vi "Teleop.vi"(10 "Match Info":T1={"Autonomous Elapsed Seconds"=0.0, "TeleOp Elapsed Seconds"=0.0, "Disabled Elapsed Seconds"=0.0, "Visited Autonomous"=FALSE, "Visited TeleOp"=FALSE, "Visited Disabled"=FALSE, "Autonomous Settings"={"Autonomous Style"=enum."Independent", "VI Refnum"=refnum}}, 11 "Call Context":T2) -> ()   [LabVIEW 2012]
doc: "This VI is called for each TeleOp packet received from the DS where the robot is not disabled. It is often used to read from the joysticks and update I/O or to update setpoints for timed control loops. It should complete and return within 20 milliseconds or it may miss DS packets."
uses:
  <vilib>/Rock Robotics/WPI/DriverStation/WPI_DriverStationDerivedRobotMode.ctl
  <vilib>/Rock Robotics/WPI/DriverStation/WPI_DriverStationMatch Info.ctl
  BotStatus.vi
  Robot Global Data.vi
  <vilib>/Rock Robotics/WPI/Joystick/WPI_JoystickGetSetRefNum.vi
  <vilib>/Rock Robotics/WPI/RobotDrive/WPI_RobotDriveGetSetRefNum.vi
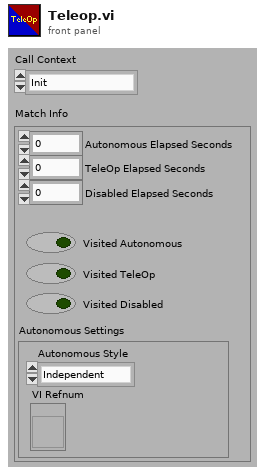
[diagram p1: front panel]
types:
  T1 = typedef "WPI_DriverStationMatch Info.ctl" = cluster{"Autonomous Elapsed Seconds":dbl, "TeleOp Elapsed Seconds":dbl, "Disabled Elapsed Seconds":dbl, "Visited Autonomous":bool, "Visited TeleOp":bool, "Visited Disabled":bool, "Autonomous Settings":cluster{"Autonomous Style":enum16{"Iterative", "Independent"}, "VI Refnum":refnum<vi>}}
  T2 = typedef "WPI_DriverStationDerivedRobotMode.ctl" = enum16{"Init", "Execute", "Stop"}
  T3 = typedef "WPI_JoystickDevRef.ctl" = cluster{"Device":T4}
  T4 = typedef "WPI_JoystickDeviceEnum.ctl" = enum16{"USB 1", "USB 2", "USB 3", "USB 4", "Kinect 1", "Kinect 2"}
  T5 = cluster{"Middle":bool, "InFlipper":bool, "Bottom":bool, "FlipperDown":bool, "Frizbee Counter":dbl}
  T6 = typedef "WPI_RobotDriveDevRef.ctl" = cluster{"DevStatus":errorcluster, "Motors[]":T7[], "Square Inputs":bool, "Max Output":dbl, "Isochronous":bool}
  T7 = typedef "WPI_MotorControlDeviceRef.ctl" = cluster{"DeviceStatus":errorcluster, "Type":enum16{"PWM", "CAN"}, "PWM":cluster{"Digital Module":T8, "PWM Channel":T9, "DeadBand":T10}, "CAN":cluster{"Device Number":u8, "Control Mode":T11, "Semaphore":T12, "Max Vout":dbl}, "Invert":bool, "TransformRef":T13, "InvTransformRef":T13}
  T8 = typedef "FPGA_TypedefDigitalModule.ctl" = enum16{"Digital Module 1", "Digital Module 2"}
  T9 = typedef "FPGA_DIOPWMChannel.ctl" = enum8{"PWM 1", "PWM 2", "PWM 3", "PWM 4", "PWM 5", "PWM 6", "PWM 7", "PWM 8", "PWM 9", "PWM 10", "Invalid"}
  T10 = typedef "WPI_PWMDeadband.ctl" = cluster{"Name":string, "maxPositivePwm":i32, "minPositivePwm":i32, "centerPwm":i32, "maxNegativePwm":i32, "minNegativePwm":i32, "angularRange":u16}
  T11 = typedef "WPI_CANJaguar_ControlMode.ctl" = enum8{"Percent VBus", "Current", "Speed", "Position", "Voltage"}
  T12 = typedef "Semaphore RefNum" = refnum<k1>
  T13 = typedef "WPI_PWMTransform_ConPane.ctl" = refnum<vi>
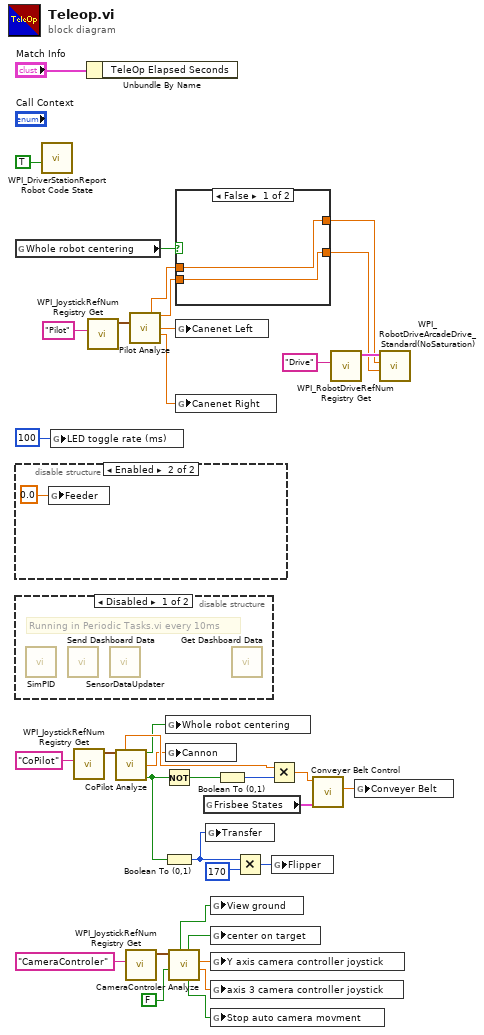
[diagram p0: block diagram]
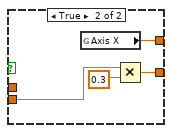
[diagram p2: hidden frame]
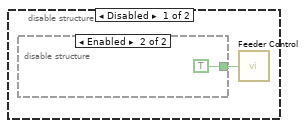
[diagram p3: hidden frame]
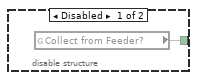
[diagram p4: hidden frame]
diagram:
  n1 = global read "BotStatus.vi" "Whole robot centering"() -> (w4:bool)
  n2 = disable-structure shown="Enabled" {
    frame Disabled {
      n3 = disable-structure shown="Enabled" {
        disable-tunnel: [w38 TRUE ("Collect from Feeder?")] -> w37
        frame Disabled {
          n4 = global read "BotStatus.vi" "Collect from Feeder?"() -> (w38)
        }
        frame Enabled {
        }
      }
      n5 = call "Feeder Control.vi"("Collect from Feeder?"=w37) -> ()  [unwired: 5 in]
    }
    frame Enabled {
      n6 = global write "BotStatus.vi" "Feeder"(0.0 ("Feeder")) -> ()
    }
  }
  n7 = disable-structure shown="Disabled" {
    frame Disabled {
      # "Running in Periodic Tasks.vi every 10ms"
      n8 = call "SimPID.vi"() -> ()  [unwired: 9 in, 2 out]
      n9 = call "Send Dashboard Data.vi"() -> ()  [unwired: 12 in]
      n10 = call "SensorDataUpdater.vi"() -> ()  [unwired: 12 in]
      n11 = call "Get Dashboard Data.vi"() -> ()  [unwired: 12 in]
    }
    frame Enabled {
    }
  }
  n12 = call <vilib>:"WPI_DriverStationReport Robot Code State.vi"("TeleOp"=TRUE ("Autonomous")) -> ()  [unwired: 10 in, 1 out]
  n13 = global write "Robot Global Data.vi" "LED toggle rate (ms)"(u32 100 ("LED ms toggle rate")) -> ()
  n14 = call <vilib>:"WPI_JoystickRefNum Registry Get.vi"("refnum name"="CoPilot") -> ("JoystickDevRef"=w28:T3)  [unwired: 1 in, 9 out]
  n15 = Unbundle By Name("Match Info") -> ()  [unwired: 1 out]
  n16 = call <vilib>:"WPI_JoystickRefNum Registry Get.vi"("refnum name"="Pilot") -> ("JoystickDevRef"=w30:T3)  [unwired: 1 in, 9 out]
  n17 = call "CoPilot Analyze.vi"("JoystickDevRef"=w28) -> ("ConveyerBelt"=w25:dbl, "Automatic fire"=w3:bool, "Shoot Motors"=w21:dbl, "La Fire at will?"=w17:bool)  [unwired: 11 in]
  n18 = call <vilib>:"WPI_JoystickRefNum Registry Get.vi"("refnum name"="CameraControler") -> ("JoystickDevRef"=w26:T3)  [unwired: 1 in, 9 out]
  n19 = call "Pilot Analyze.vi"("JoystickDevRef"=w30) -> ("x"=w5:dbl, "y"=w8:dbl, "Canenet L"=w23:dbl, "Canenet R"=w22:dbl)  [unwired: 9 in, 2 out]
  n20 = Not(x=w17) -> (.not. x?=w15:bool)
  n21 = Boolean To (0,1)(Boolean=w17) -> (0, 1=w18:i16)
  n22 = global write "BotStatus.vi" "Whole robot centering"(w3) -> ()
  n23 = global write "BotStatus.vi" "Cannon"(w21) -> ()
  n24 = call "CameraControler Analyze.vi"("Climbing Manual Enabled"=FALSE, "JoystickDevRef"=w26) -> ("axis 3 (rotation)"=w1:dbl, "Y"=w2:dbl, "stop auto camera movement"=w11:bool, "Center on Target"=w10:bool, "View Ground"=w9:bool)  [unwired: 5 in]
  n25 = case shown="False" w4 {
    tunnel: w8 -> [w42 w45]
    tunnel: [w42 w43] -> w7
    tunnel: [w41 w46] -> w6
    tunnel: w5 -> [w41 _]
    frame False {
    }
    frame True {
      n26 = global read "BotStatus.vi" "Axis X"() -> (w46:dbl)
      n27 = Multiply(x=w45, y=0.3) -> (x*y=w43:dbl)
    }
  }
  n28 = global write "BotStatus.vi" "Canenet Left"(w23) -> ()
  n29 = global write "BotStatus.vi" "Canenet Right"(w22) -> ()
  n30 = global read "BotStatus.vi" "Frisbee States"() -> (w14:T5)
  n31 = global write "BotStatus.vi" "Transfer"(w18) -> ()
  n32 = global write "BotStatus.vi" "View ground"(w9) -> ()
  n33 = global write "BotStatus.vi" "center on target"(w10) -> ()
  n34 = global write "BotStatus.vi" "Y axis camera controller joystick"(w2) -> ()
  n35 = global write "BotStatus.vi" "axis 3 camera controller joystick"(w1) -> ()
  n36 = global write "BotStatus.vi" "Stop auto camera movment"(w11) -> ()
  n37 = Boolean To (0,1)(Boolean=w15) -> (0, 1=w16:i16)
  n38 = Multiply(x=w18, y=i16 170 ("0, 1")) -> (x*y=w20:i16)
  n39 = Multiply(x=w25, y=w16) -> (x*y=w12:dbl)
  n40 = global write "BotStatus.vi" "Flipper"(w20) -> ()
  n41 = call "Conveyer Belt Control.vi"("Frisbee States"=w14, "conveyer belt control"=w12) -> ("conveyer belt"=w13:dbl)  [unwired: 9 in]
  n42 = call <vilib>:"WPI_RobotDriveRefNum Registry Get.vi"("refnum name"="Drive") -> ("RobotDriveDevRef"=w34:T6)  [unwired: 1 in, 9 out]
  n43 = global write "BotStatus.vi" "Conveyer Belt"(w13) -> ()
  n44 = call <vilib>:"WPI_RobotDriveArcadeDrive_Standard(NoSaturation).vi"("Y axis value"=w7, "X axis value"=w6, "RobotDriveDevRef"=w34) -> ()  [unwired: 1 in, 8 out]
